vi "ProcessHealthAndStatusUpdates.vi"(10 "healthAndStatusMemory":refnum<k21>="HealthAndStatusMemory", 11 "internalHealthAndStatusFIFO":refnum<k21>="InternalHealthAndStatusFIFO") -> ()   [LabVIEW 2015, in "FPGAHealthAndStatus.lvlib"]
uses:
  FPGAHealthAndStatus.lvlib
  <vilib>/rvi/Emulation/niFpgaGetClockAttributes.vi
  <vilib>/rvi/Emulation/niFpgaSctlEmulationGetInTimedLoop.vi
  <vilib>/rvi/Emulation/niFpgaEmulationReportErrorSimple.vi
  <vilib>/rvi/DataTransferAndStorage/Container/Common/niFpgaContainerExecOnDevCompGetState.vi
  <vilib>/rvi/Emulation/niFpgaEmulationIsFPGAContextNoSignature.vi
  <vilib>/rvi/errors/niFpgaSetErrorForExecOnDevCompSimple.vi
  <vilib>/rvi/eio/common/nirviEmuReportErrorAndStop.vi
  <vilib>/rvi/DataTransferAndStorage/Container/Common/niFpgaContainerGetUniqueNameForEmu.vi
  <vilib>/rvi/FIFO/Fifo_Resource/nirvififoEmulationSetSize.vi
  <vilib>/rvi/FIFO/Fifo_Resource/nirviFifoEmulationQueueMgr.vi
  <instcachedir>/0/nirviFifoEmulationQueueMgr_E5CAEC123FF24DC58D834DCA3CDAA9B5.lvgen/nirviFifoEmulationQueueMgr_E5CAEC123FF24DC58D834DCA3CDAA9B5_008.vi
  <vilib>/rvi/FIFO/Fifo_Resource/nirvififoEmulationDetermineInputValidOut.vi
  <vilib>/rvi/FIFO/Fifo_Resource/nirvififoEmulationCreateLock.vi
  <vilib>/rvi/Emulation/niFpgaProcessEmulError.vi
  <vilib>/rvi/FIFO/Fifo_Resource/nirvififoEmulationObtainLock.vi
  <vilib>/rvi/FIFO/Fifo_Resource/nirvififoEmulationReleaseLock.vi
  <vilib>/rvi/occurrence/nirviWaitOnOccurrenceBase.vi
  <vilib>/rvi/errors/nirviReportUnexpectedCaseInternalError.vi
  <vilib>/rvi/errors/nirviReportUnexpectedCaseInternalError (U32).vi
  <vilib>/Utility/error.llb/Clear Errors.vi
  <vilib>/rvi/interface/RandomDataEmulation/niFpgaRandomDataHandleErrors.vi
  <vilib>/rvi/Memory/Memory_Emulation/niFpgaMemoryEmulationCacheClearOnFirstRun.vi
  <vilib>/rvi/Memory/Memory_Emulation/nirvimemoryEmulationManagerCache_MakeExclusive.vi
  <vilib>/rvi/Memory/Memory_Emulation/niFpgaMemoryEmulationValidateCache.vi
  <vilib>/rvi/Memory/Memory_Emulation/nirvimemoryEmulationManagerCache_InsertValue.vi
  <vilib>/rvi/Memory/Memory_Emulation/nirvimemoryEmulationManagerCache_ReleaseExclusive.vi
  <vilib>/rvi/Memory/Memory_Emulation/nirvimemoryEmulationManagerCache_GetValue.vi
  <vilib>/rvi/Memory/Memory_Emulation/nirvimemoryEmulationManagerCache_SetValue.vi
  <vilib>/rvi/Emulation/niFpgaSctlEmulationResourceMgr.vi
  <vilib>/rvi/Emulation/niFpgaCriticalErrorInLSC.vi
  <vilib>/rvi/DataTransferAndStorage/Container/XNode/niFpgaContainer.xnode
  <vilib>/rvi/FIFO/Fifo_Resource/niFpgaFifoEmulationRefIn.vi
  <vilib>/rvi/Memory/Memory_Emulation/niFpgaMemoryEmulationRefIn.vi
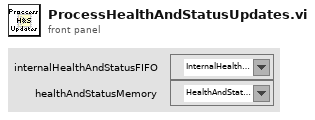
[diagram p1: front panel]
types:
  T1 = cluster{"Address":u32, "Telemetry Update Mode":enum8{"NOP", "Set", "Add", "Subtract", "Or"}, "Data":u32}
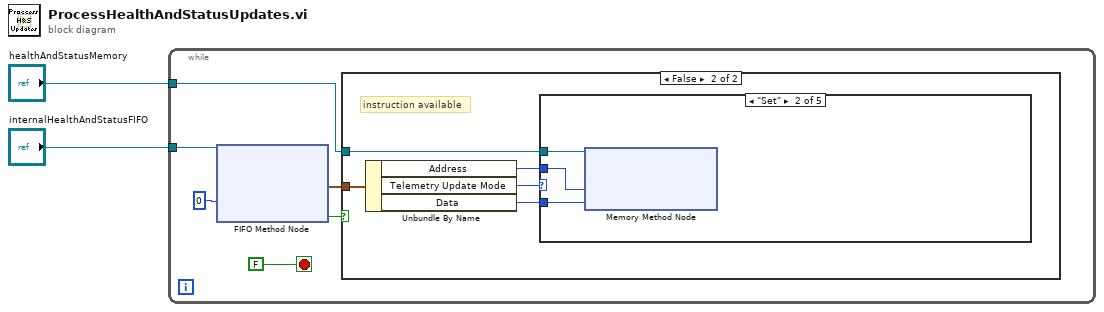
[diagram p0: block diagram]
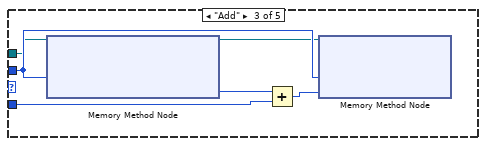
[diagram p4: hidden frame]
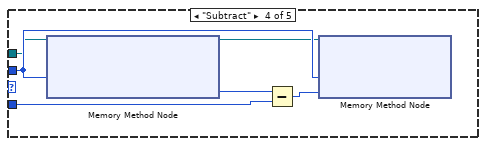
[diagram p5: hidden frame]
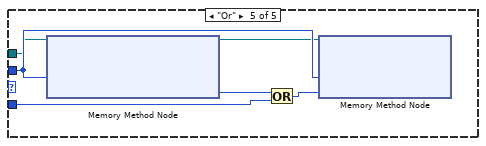
[diagram p6: hidden frame]
diagram:
  n1 = while {
    tunnel: "internalHealthAndStatusFIFO" -> [w4]
    tunnel: "healthAndStatusMemory" -> [w3]
    stop <- FALSE stop-if-true
    n2 = xnode ("FIFO Method Node")("Timeout"=0, "FIFO In"=w4) -> ("Element"=w6:T1, "Timed Out?"=w7:bool)  [unwired: 1 out]
    n3 = case shown="False" w7 {
      tunnel: w6 -> [_ w13]
      tunnel: w3 -> [_ w9]
      frame True {
        # "no instruction available"
      }
      frame False {
        # "instruction available"
        n4 = Unbundle By Name(w13) -> ("Address"=w11:u32, "Telemetry Update Mode"=w12:enum8{"NOP", "Set", "Add", "Subtract", "Or"}, "Data"=w10:u32)
        n5 = case shown="\"Set\"" w12 {
          tunnel: w11 -> [_ w16 w21 w27 w33]
          tunnel: w10 -> [_ w15 w19 w25 w31]
          tunnel: w9 -> [_ w14 w18 w24 w30]
          frame "NOP", Default {
          }
          frame "Set" {
            n6 = xnode ("Memory Method Node")("Address"=w16, "Data"=w15, "Memory In"=w14) -> ()  [unwired: 1 out]
          }
          frame "Add" {
            n7 = xnode ("Memory Method Node")("Address"=w21, "Memory In"=w18) -> ("Data"=w22:u32, "Memory Out"=w17:refnum<k21>)
            n8 = Add(x=w22, y=w19) -> (x+y=w20:u32)
            n9 = xnode ("Memory Method Node")("Address"=w21, "Data"=w20, "Memory In"=w17) -> ()  [unwired: 1 out]
          }
          frame "Subtract" {
            n10 = xnode ("Memory Method Node")("Address"=w27, "Memory In"=w24) -> ("Data"=w28:u32, "Memory Out"=w23:refnum<k21>)
            n11 = Subtract(x=w28, y=w25) -> (x-y=w26:u32)
            n12 = xnode ("Memory Method Node")("Address"=w27, "Data"=w26, "Memory In"=w23) -> ()  [unwired: 1 out]
          }
          frame "Or" {
            n13 = xnode ("Memory Method Node")("Address"=w33, "Memory In"=w30) -> ("Data"=w34:u32, "Memory Out"=w29:refnum<k21>)
            n14 = Or(x=w34, y=w31) -> (x .or. y?=w32:u32)
            n15 = xnode ("Memory Method Node")("Address"=w33, "Data"=w32, "Memory In"=w29) -> ()  [unwired: 1 out]
          }
        }
      }
    }
  }
